vi "Eth Status Read Start.vi"(8 "error in (no error)":errorcluster, 9 "timeout (0)":i32, 11 "Set_state":refnum<queue>) -> (0 "error out":errorcluster, 1 "Stop":bool, 2 "Start":bool, 3 "Set_state out":refnum<queue>, 4 "timed out?":bool)   [LabVIEW 2021, in "Eth Status.lvlib"]
uses:
  Eth Status.lvlib
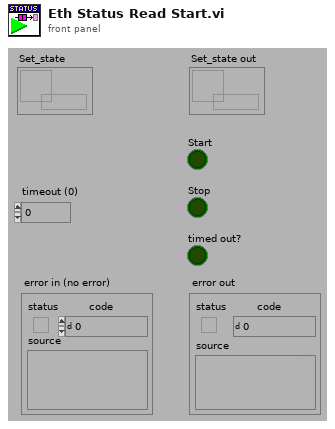
[diagram p1: front panel]
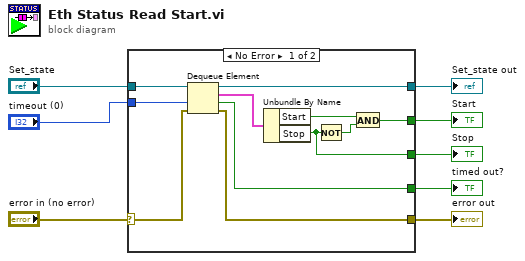
[diagram p0: block diagram]
diagram:
  n1 = case shown="No Error" "error in (no error)" {
    selector: "error in (no error)" -> [w17 w21]
    tunnel: [w12 w21] -> w8
    tunnel: [w13 _] -> w6
    tunnel: "timeout (0)" -> [w18 _]
    tunnel: "Set_state" -> [w19 w20]
    tunnel: [w11 w20] -> w1
    tunnel: [w10 _] -> w4
    tunnel: [w9 _] -> w3
    frame No Error {
      n2 = Dequeue Element(queue=w19, timeout in ms (-1)=w18, error in (no error)=w17) -> (queue out=w11:refnum<queue>, element=w16:cluster{"Start":bool, "Stop":bool}, timed out?=w10:bool, error out=w12:errorcluster)
      n3 = Unbundle By Name(w16) -> ("Start"=w15:bool, "Stop"=w9:bool)
      n4 = Not(x=w9) -> (.not. x?=w14:bool)
      n5 = And(x=w15, y=w14) -> (x .and. y?=w13:bool)
    }
    frame Error {
    }
  }
  "error out" <- w8
  "Start" <- w6
  "timed out?" <- w4
  "Stop" <- w3
  "Set_state out" <- w1
